vi "sample8(DXL).vi"() -> ()   [LabVIEW 2020]
panel:
  out "mon_ok":bool
  in  "OffsetTime":u32=500
  out "ModelInfo":T1
  out "rpm":dbl
  out "current":dbl
  out "angle":dbl
  out "success":bool
  in  "mode":u8(ring)=3 items=["OpCurrent"=0, "OpVelocity"=1, "OpPosition"=3, "OpExPosition"=4, "OpCurExPosition"=5, "OpPWM"=16]
  out "ErrorCode":u16 format="%04x"
  in  "ID":u8=1 max=253
  in  "Baudrate":u32=57600 min=9600 max=12000000
  in  "COM":refnum<visa-resource-name> caption="COMポート"
  in  "STOP":bool
  in  "Value":dbl(knob) scale=720.0..-720.0
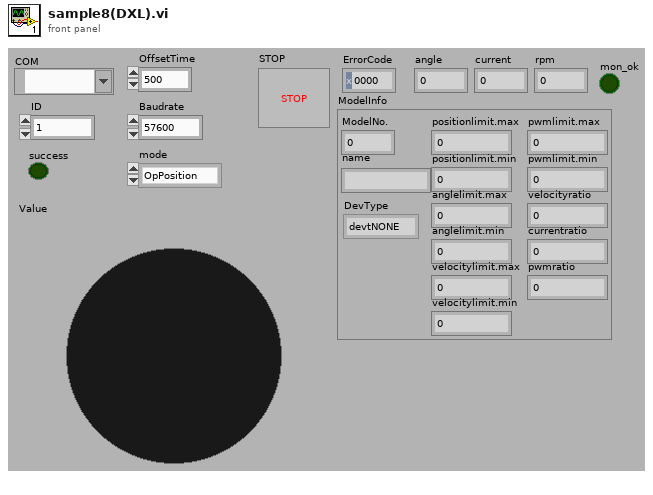
[diagram p1: front panel]
types:
  T1 = cluster{"ModelNo.":u16, "name":string, "DevType":enum32{"devtNONE", "devtDX", "devtAX", "devtRX", "devtEX", "devtMX", "devtXL320", "devtPRO", "devtX"}, "positionlimit.max":i32, "positionlimit.min":i32, "anglelimit.max":dbl, "anglelimit.min":dbl, "velocitylimit.max":i32, "velocitylimit.min":i32, "pwmlimit.max":i32, "pwmlimit.min":i32, "velocityratio":dbl, "currentratio":dbl, "pwmratio":dbl}
  T2 = enum32{"devtNONE", "devtDX", "devtAX", "devtRX", "devtEX", "devtMX", "devtXL320", "devtPRO", "devtX"}
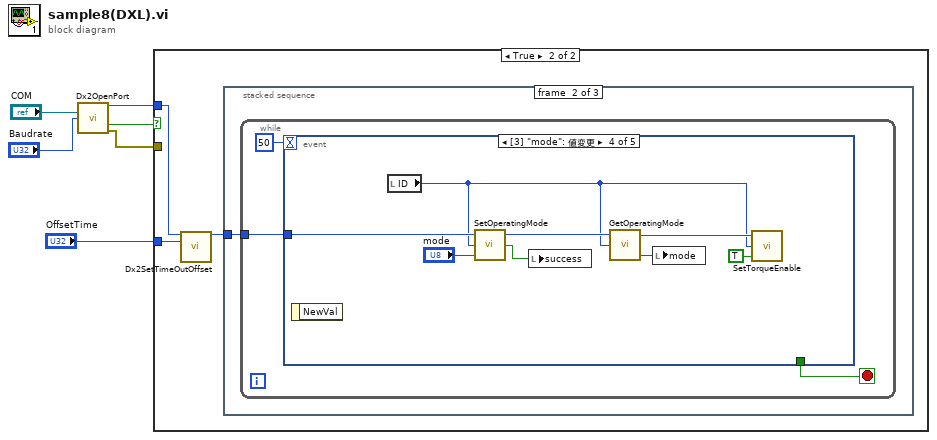
[diagram p0: block diagram]
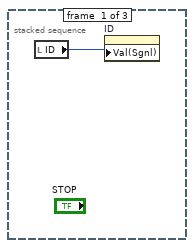
[diagram p3: hidden frame]
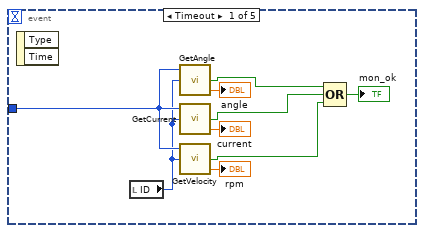
[diagram p4: hidden frame]
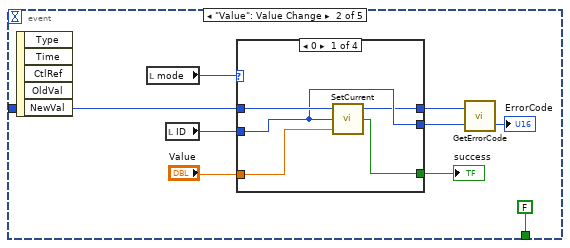
[diagram p5: hidden frame]
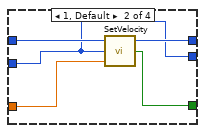
[diagram p6: hidden frame]
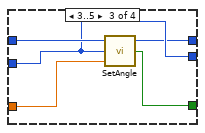
[diagram p7: hidden frame]
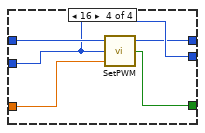
[diagram p8: hidden frame]
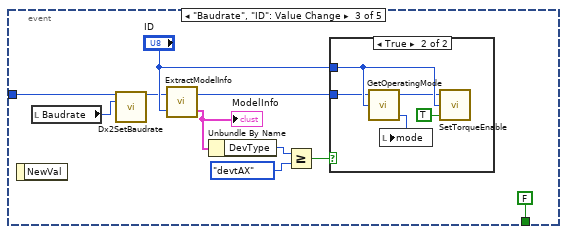
[diagram p9: hidden frame]
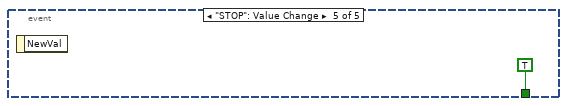
[diagram p11: hidden frame]
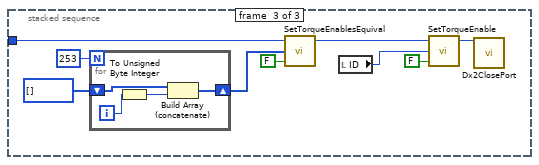
[diagram p12: hidden frame]
diagram:
  n1 = call "Dx2OpenPort.vi"("port"="COM", "baudrate"="Baudrate") -> ("dvid"=w4:u32, "成功"=w3:bool, "エラー出力"=w2:errorcluster)  [unwired: 11 in]
  n2 = case shown="TRUE" w3 {
    tunnel: w4 -> [_ w7]
    tunnel: w2 -> [_ _]
    tunnel: "OffsetTime" -> [_ w9]
    frame False {
    }
    frame True {
      n3 = call "Dx2SetTimeOutOffset.vi"("dvid in"=w7, "OffsetTime"=w9) -> ("dvid out"=w8:u32)  [unwired: 12 in, 1 out]
      n4 = stacked-sequence {
        tunnel: w8 -> [_ w11 w78]
        frame #0 {
          n5 = local read "ID"() -> (w10:u8)
          n6 = property on="ID" class="DigNum (指定)"("Val(Sgnl)"=w10) -> ()  [unwired: 2 in, 2 out]
        }
        frame #1 {
          n7 = while {
            tunnel: w11 -> [w13]
            stop <- w12 stop-if-true
            n8 = event shown="[3] \"mode\": 値変更" {
              selector: _ -> [_ _ _ _ _]
              dyn-events: _ -> [_ _ _ _ _]
              timeout: 50 -> [_ _ _ _ _]
              tunnel: w13 -> [w23 w30 w54 w74 _]
              tunnel: [_ FALSE FALSE _ TRUE] -> w12
              event Timeout {
                n9 = event-data() -> ()  [unwired: 1 in, 2 out]
                n10 = local read "ID"() -> (w22:u8)
                n11 = call "GetAngle.vi"("Target ID"=w22, "dvid in"=w23) -> ("angle"=→"angle":dbl, "success"=w18:bool)  [unwired: 1 in, 1 out]
                n12 = call "GetCurrent.vi"("Target ID"=w22, "dvid in"=w23) -> ("current"=→"current":dbl, "success"=w17:bool)  [unwired: 1 in, 1 out]
                n13 = call "GetVelocity.vi"("Target ID"=w22, "dvid in"=w23) -> ("velocity"=→"rpm":dbl, "success"=w16:bool)  [unwired: 1 in, 1 out]
                n14 = Compound Arithmetic op=OR ("複合演算")(w18, w17, w16) -> (→"mon_ok":bool)
              }
              event "Value": Value Change {
                n15 = event-data() -> ()  [unwired: 1 in, 5 out]
                n16 = local read "mode"() -> (w31:u8)
                n17 = local read "ID"() -> (w29:u8)
                n18 = case shown="0" w31 {
                  tunnel: w30 -> [w37 w42 w47 w52]
                  tunnel: w29 -> [w36 w40 w46 w51]
                  tunnel: [w35 w41 w45 w49] -> w27
                  tunnel: [w36 w40 w46 w51] -> w26
                  tunnel: "Value" -> [w34 w39 w44 w50]
                  tunnel: [w33 w38 w43 w48] -> w24
                  frame 0 {
                    n19 = call "SetCurrent.vi"("current"=w34, "Target ID"=w36, "dvid in"=w37) -> ("success"=w33:bool, "dvid out"=w35:u32)  [unwired: 1 in]
                  }
                  frame 1, Default {
                    n20 = call "SetVelocity.vi"("velocity"=w39, "Target ID"=w40, "dvid in"=w42) -> ("success"=w38:bool, "dvid out"=w41:u32)  [unwired: 1 in]
                  }
                  frame 3..5 {
                    n21 = call "SetAngle.vi"("angle"=w44, "Target ID"=w46, "dvid in"=w47) -> ("success"=w43:bool, "dvid out"=w45:u32)  [unwired: 1 in]
                  }
                  frame 16 {
                    n22 = call "SetPWM.vi"("PWM"=w50, "Target ID"=w51, "dvid in"=w52) -> ("success"=w48:bool, "dvid out"=w49:u32)  [unwired: 1 in]
                  }
                }
                "success" <- w24
                n23 = call "GetErrorCode.vi"("Target ID"=w26, "dvid in"=w27) -> ("ErrorCode"=→"ErrorCode":u16)  [unwired: 1 out]
              }
              event "Baudrate", "ID": Value Change {
                n24 = event-data() -> ()  [unwired: 1 in, 1 out]
                n25 = local read "Baudrate"() -> (w55:u32)
                n26 = call "Dx2SetBaudrate.vi"("dvid in"=w54, "Baudrate"=w55) -> ("dvid out"=w53:u32)  [unwired: 11 in, 2 out]
                n27 = call "ExtractModelInfo.vi"("Target ID"="ID", "dvid in"=w53) -> ("ModelInfo"=w60:T1, "dvid out"=w62:u32)
                "ModelInfo" <- w60
                n28 = Unbundle By Name(w60) -> ("DevType"=w59:T2)
                n29 = Greater Or Equal?(x=w59, y=T2."devtAX" ("DevType")) -> (x >= y?=w57:bool)
                n30 = case shown="TRUE" w57 {
                  tunnel: w62 -> [_ w63]
                  tunnel: "ID" -> [_ w67]
                  frame False {
                  }
                  frame True {
                    n31 = call "GetOperatingMode.vi"("Target ID"=w67, "dvid in"=w63) -> ("mode"=w64:u8, "dvid out"=w65:u32)  [unwired: 1 in, 1 out]
                    n32 = local write "mode"(w64) -> ()
                    n33 = call "SetTorqueEnable.vi"("torqueenable"=TRUE, "Target ID"=w67, "dvid in"=w65) -> ()  [unwired: 1 in, 2 out]
                  }
                }
              }
              event "mode": Value Change {
                n34 = event-data() -> ()  [unwired: 1 in, 1 out]
                n35 = local read "ID"() -> (w68:u8)
                n36 = call "SetOperatingMode.vi"("mode"="mode", "Target ID"=w68, "dvid in"=w74) -> ("success"=w71:bool, "dvid out"=w72:u32)  [unwired: 1 in]
                n37 = local write "success"(w71) -> ()
                n38 = call "GetOperatingMode.vi"("Target ID"=w68, "dvid in"=w72) -> ("mode"=w73:u8, "dvid out"=w69:u32)  [unwired: 1 in, 1 out]
                n39 = local write "mode"(w73) -> ()
                n40 = call "SetTorqueEnable.vi"("torqueenable"=TRUE, "Target ID"=w68, "dvid in"=w69) -> ()  [unwired: 1 in, 2 out]
              }
              event "STOP": Value Change {
                n41 = event-data() -> ()  [unwired: 1 in, 1 out]
              }
            }
          }
        }
        frame #2 {
          n42 = for {
            N: 253 -> [_]
            shift-right: [w88] -> w80
            shift-left: u8[] [] -> [w89]
            i -> [w87]
            n43 = To Unsigned Byte Integer(number=w87) -> (unsigned 8bit integer=w86:u8)
            n44 = Build Array (concatenate)(w89, w86) -> (w88:u8[])
          }
          n45 = call "SetTorqueEnablesEquival.vi"("torqueenable"=FALSE, "ids"=w80, "dvid in"=w78) -> ("dvid out"=w77:u32)  [unwired: 1 in, 1 out]
          n46 = local read "ID"() -> (w83:u8)
          n47 = call "SetTorqueEnable.vi"("torqueenable"=FALSE, "Target ID"=w83, "dvid in"=w77) -> ("dvid out"=w85:u32)  [unwired: 1 in, 1 out]
          n48 = call "Dx2ClosePort.vi"("dvid"=w85) -> ()  [unwired: 13 in, 2 out]
        }
      }
    }
  }
